vi "Batch Retrieve External Sensors.vi"(9 "Include Volts":T1, 11 "Hold Data":T1) -> (2 "Data":dbl[](array[numeric]))   [LabVIEW 2009]
uses:
  Apps/Yes No Button.ctl
  Dataset Transaction Id.ctl
  Dataset Source.ctl
  Dataset Type.ctl
  Data Access Objects/Metadata/DAO Actions.ctl
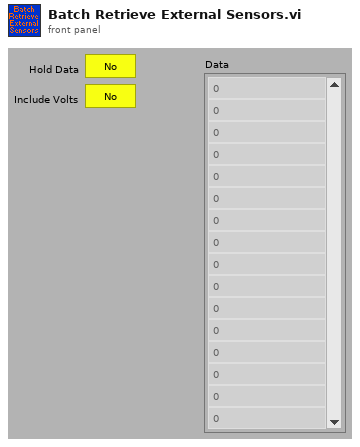
[diagram p1: front panel]
types:
  T1 = typedef "Yes No Button.ctl" = bool
  T2 = typedef "Dataset Type.ctl" = enum16{"LVDT", "Load Cell", "Actuator Command", "Servo Error", "Displacement Command", "Displacement", "Force"}
  T3 = typedef "Dataset Source.ctl" = enum16{"LBCB 1", "LBCB 2", "Combined", "External Sensors"}
  T4 = typedef "Dataset Transaction Id.ctl" = cluster{"Dataset Source":T3, "Dataset Type":T2, "Hold":T1, "Volts":T1, "Tag":string}
  T5 = typedef "DAO Actions.ctl" = enum16{"Init", "Get", "Set"}
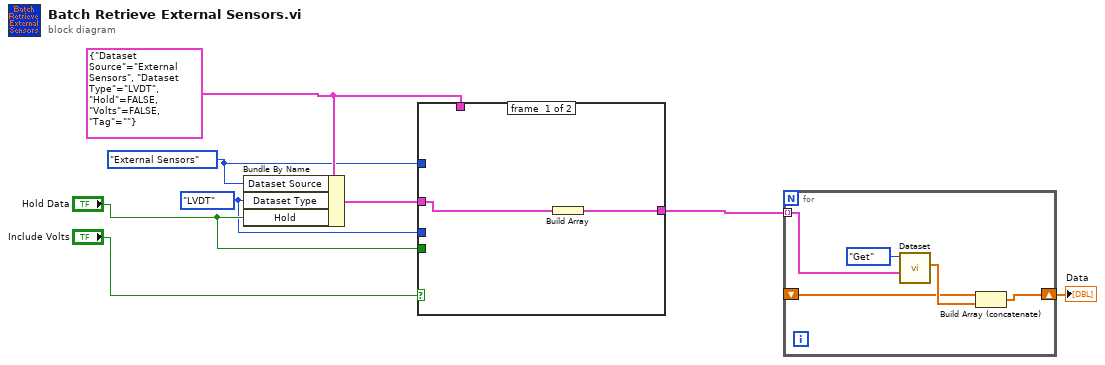
[diagram p0: block diagram]
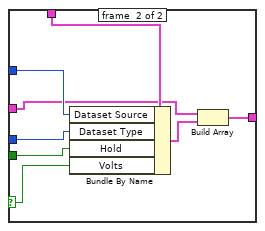
[diagram p2: hidden frame]
diagram:
  w3 = Dataset_Type."LVDT" ("Dataset Type")
  w4 = Dataset_Source."External Sensors" ("Dataset Source")
  w6 = T4 {"Dataset Source"=enum."External Sensors", "Dataset Type"=enum."LVDT", "Hold"=FALSE, "Volts"=FALSE, "Tag"=""} ("Dataset Trans Id")
  n1 = Bundle By Name(cluster=w6, "Dataset Source"=w4, "Dataset Type"=w3, "Hold"="Hold Data") -> (w7:T4)
  n2 = case shown="False" "Include Volts" {
    selector: "Include Volts" -> [_ w13]
    tunnel: w7 -> [w10 w12]
    tunnel: w6 -> [_ w18]
    tunnel: "Hold Data" -> [_ w17]
    tunnel: w4 -> [_ w16]
    tunnel: w3 -> [_ w15]
    tunnel: [w9 w11] -> w2
    frame #0 {
      n3 = Build Array(w10) -> (w9:T4[])
    }
    frame #1 {
      n4 = Bundle By Name(cluster=w18, "Dataset Source"=w16, "Dataset Type"=w15, "Hold"=w17, "Volts"=w13) -> (w14:T4)
      n5 = Build Array(w12, w14) -> (w11:T4[])
    }
  }
  n6 = for {
    tunnel: w2 -> [w23] mode=indexing
    shift-right: [w20] -> w1
    shift-left: _ -> [w19]
    n7 = call "Dataset.vi"("Dataset Trans Id"=w23, "DAO Actions"=DAO_Actions."Get") -> ("Data Out"=w21:dbl[])  [unwired: 8 in, 1 out]
    n8 = Build Array (concatenate)(w19, w21) -> (w20:dbl[])
  }
  "Data" <- w1
